vi "Avg_ChirpV2.vi"(11 "Array":dbl[](array[numeric])) -> (3 "Avg":dbl)   [LabVIEW 2014]
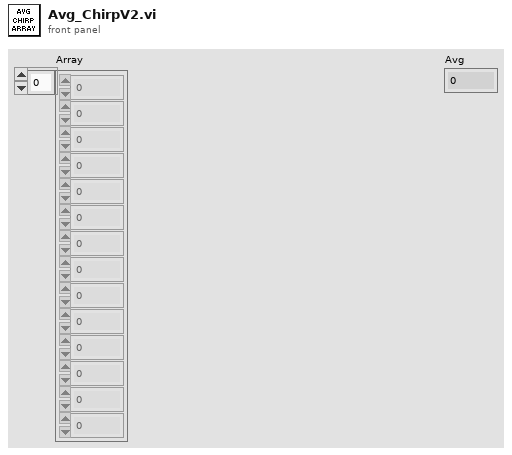
[diagram p1: front panel]
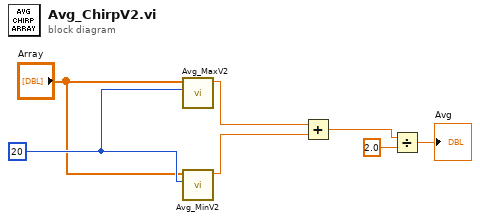
[diagram p0: block diagram]
diagram:
  w7 = 20 ("# of Max")
  n1 = call "Avg_MaxV2.vi"("# of Max"=w7, "Array"="Array") -> ("Avg Max"=w5:dbl)  [unwired: 9 in]
  n2 = call "Avg_MinV2.vi"("# of Min"=w7, "Array"="Array") -> ("Avg Min"=w4:dbl)  [unwired: 9 in]
  n3 = Add(x=w5, y=w4) -> (x+y=w3:dbl)
  n4 = Divide(x=w3, y=2.0) -> (x/y=→"Avg":dbl)
